vi "Read Teller.vi"(11 "Stopping Msg Input in":refnum<class "Stopping Msg Input.lvclass">) -> (2 "Teller":T1 {"Time" format="%<%x %.3X>T"})   [LabVIEW 2020, in "jettl.lvlib" / "Stopping jettl Msg.lvlib" / "Stopping Msg Input.lvlib" / "Stopping Msg Input.lvclass"]
doc: "jettl 6.12.1.94\nNathan Davis - Nathan Davis\nCopyright (c) 2026, Nathan Davis\nMIT"
uses:
  Stopping Msg Input.lvclass
  Stopping Msg Input.lvclass/Stopping Msg Input.ctl
  Relation.ctl
  jettl.lvlib
  Teller Metadata/Teller Metadata.lvclass
  Teller.ctl
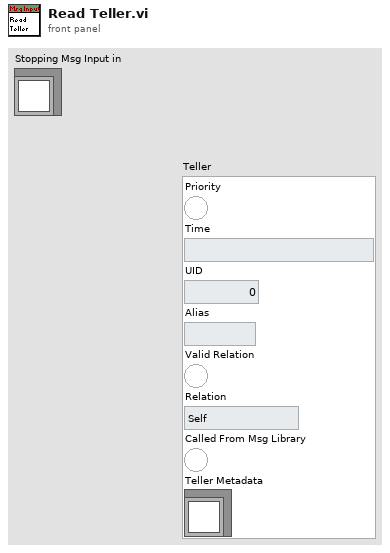
[diagram p1: front panel]
types:
  T1 = typedef "jettl.lvlib/Teller.ctl" = cluster{"Priority":bool, "Time":timestamp, "UID":i32, "Alias":string, "Valid Relation":bool, "Relation":T2, "Called From Msg Library":bool, "Teller Metadata":refnum<class "Teller Metadata.lvclass">}
  T2 = typedef "jettl.lvlib/Relation.ctl" = enum16{"Self", "Parent", "Child"}
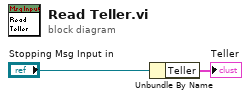
[diagram p0: block diagram]
diagram:
  n1 = Unbundle By Name("Stopping Msg Input in") -> ("Teller"=→"Teller":T1)
